vi "S2C_PCIe7841_Proc_DigitalWrite.vi"(8 "Error In":errorcluster, 11 "Data":string) -> (0 "Error Out":errorcluster)   [LabVIEW 2015]
uses:
  S2C_PCIe7841_Proc_Globals.vi
  <vilib>/Utility/error.llb/Error Cluster From Error Code.vi
  <vilib>/rvi/errors/niLvFpgaAdjustHostInterfaceError.vi
  <vilib>/rvi/interface/nirviMethod/nirviMethod.xnode
  <vilib>/FPGAPlugInAG/Dynamic/niLvFpga_WriteFifo_Dynamic.vi
  <vilib>/rvi/errors/niLvFpgaMergeErrorWithErrorCode.vi
panel:
  out "Conn":u8
  out "Data":u16 format="%016b"
  out "Size":bool
  out "State":bool
  out "Port":bool[](array[boolean])
  out "Bits":bool[](array[boolean])
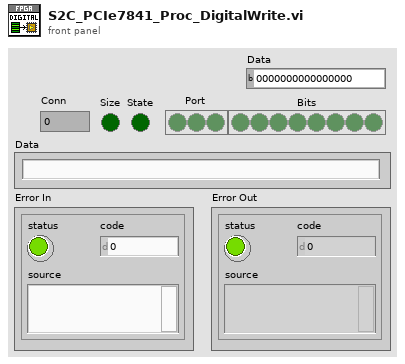
[diagram p1: front panel]
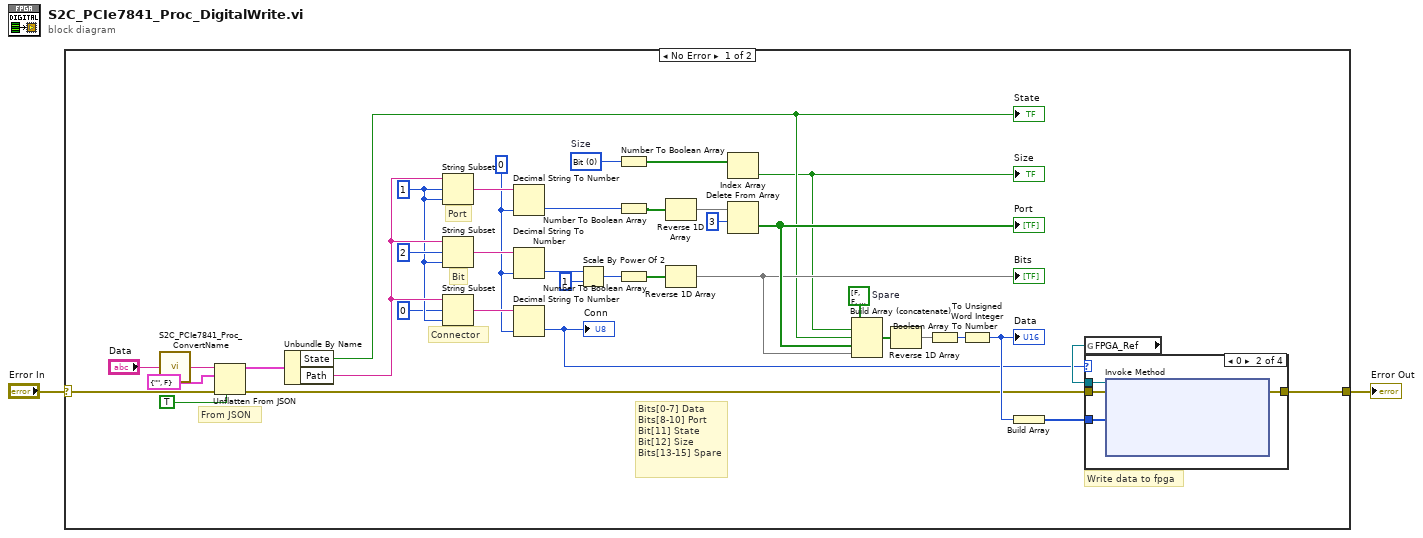
[diagram p0: block diagram]
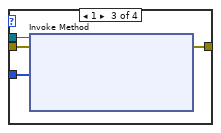
[diagram p3: hidden frame]
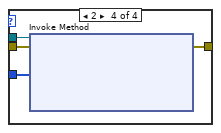
[diagram p4: hidden frame]
diagram:
  n1 = case shown="No Error" "Error In" {
    selector: "Error In" -> [w40 w54]
    tunnel: [w18 w54] -> w1
    frame No Error {
      w11 = u8 0 items=["Bit", "Port"]  # Size
      w27 = bool[] [FALSE, FALSE, FALSE, FALSE]  # Spare
      w29 = u8 0
      w14 = 1 ("offset (0)")
      # "Bits[0-7] Data\nBits[8-10] Port\nBit[11] State\nBit[12] Size\nBits[13-15] Spare"
      # "Port"
      # "Bit"
      # "Connector"
      # "Write data to fpga"
      # "From JSON"
      n2 = call "S2C_PCIe7841_Proc_ConvertName.vi"("Data In"="Data") -> ("Data Out"=w3:string)  [unwired: 4 in]
      n3 = Unflatten From JSON(JSON string=w3, type and defaults=cluster{"Path":string, "State":bool} {"Path"="", "State"=FALSE}, default null elements? (F)=TRUE, error in (no error)=w40) -> (value=w38:cluster{"Path":string, "State":bool}, error out=w15:errorcluster)  [unwired: 3 in]
      n4 = Unbundle By Name(w38) -> ("State"=w9:bool, "Path"=w16:string)
      "State" <- w9
      n5 = String Subset(string=w16, offset (0)=w14, length (rest)=w14) -> (substring=w35:string)
      n6 = String Subset(string=w16, offset (0)=2, length (rest)=w14) -> (substring=w34:string)
      n7 = String Subset(string=w16, offset (0)=0, length (rest)=w14) -> (substring=w36:string)
      n8 = Decimal String To Number(string=w35, default (0L)=w29) -> (number=w6:u8)  [unwired: 1 in, 1 out]
      n9 = Decimal String To Number(string=w34, default (0L)=w29) -> (number=w33:u8)  [unwired: 1 in, 1 out]
      n10 = Decimal String To Number(string=w36, default (0L)=w29) -> (number=w7:u8)  [unwired: 1 in, 1 out]
      "Conn" <- w7
      n11 = Scale By Power Of 2(n=w33, x=u8 1) -> (x*2^n=w5:u8)
      n12 = Number To Boolean Array(number=w11) -> (Boolean array=w10:bool[])
      n13 = Number To Boolean Array(number=w6) -> (Boolean array=w31:bool[])
      n14 = Number To Boolean Array(number=w5) -> (Boolean array=w32:bool[])
      n15 = Reverse 1D Array(array=w31) -> (reversed array=w30:bool[])
      n16 = Reverse 1D Array(array=w32) -> (reversed array=w21:bool[])
      "Bits" <- w21
      n17 = Index Array(array=w10) -> (element=w8:bool)  [unwired: 1 in]
      "Size" <- w8
      n18 = Delete From Array(array=w30, length=3) -> (deleted portion=w22:bool[])  [unwired: 1 in, 1 out]
      "Port" <- w22
      n19 = Build Array (concatenate)(w27, w8, w9, w22, w21) -> (w26:bool[])
      n20 = Reverse 1D Array(array=w26) -> (reversed array=w24:bool[])
      n21 = Boolean Array To Number(Boolean array=w24) -> (number=w25:u32)
      n22 = To Unsigned Word Integer(number=w25) -> (unsigned 16bit integer=w20:u16)
      "Data" <- w20
      n23 = Build Array(w20) -> (w19:u16[])
      n24 = global read "S2C_PCIe7841_Proc_Globals.vi" "FPGA_Ref"() -> (w12:refnum<k20>)
      n25 = case shown="0" w7 {
        tunnel: w15 -> [w41 w45 w49 w53]
        tunnel: w19 -> [_ w44 w48 w52]
        tunnel: [w41 w43 w47 w51] -> w18
        tunnel: w12 -> [_ w42 w46 w50]
        frame 4, Default {
        }
        frame 0 {
          n26 = xnode "Invoke Method"("FPGA VI Reference In"=w42, "error in"=w45, "Data"=w44) -> ("error out"=w43:errorcluster)  [unwired: 1 in, 2 out]
        }
        frame 1 {
          n27 = xnode "Invoke Method"("FPGA VI Reference In"=w46, "error in"=w49, "Data"=w48) -> ("error out"=w47:errorcluster)  [unwired: 1 in, 2 out]
        }
        frame 2 {
          n28 = xnode "Invoke Method"("FPGA VI Reference In"=w50, "error in"=w53, "Data"=w52) -> ("error out"=w51:errorcluster)  [unwired: 1 in, 2 out]
        }
      }
    }
    frame Error {
    }
  }
  "Error Out" <- w1
